vi "Read alarm XML.vi"(11 "模块名称":string) -> (3 "报警输出":string[][](array[string]))   [LabVIEW 2016, in "斯坦道CODMn新电路板.lvlib"]
uses:
  <vilib>/Utility/xml.llb/Write to XML File(string).vi
  <vilib>/Utility/xml.llb/Read From XML File(string).vi
panel:
  in  "报警常量":string[][](array[string])=[["1", "1007", "缺试剂告警", "1、是否缺试剂，及时补充试剂\n2、对应的试剂阀口堵塞，及时清理并更换连接头。\n3、管路气密性不佳\n4、检查传感器与电路板连接、查看传感器光值是否异常"], ["2", "1008", "缺水样告警", "1、配水箱内无水样\n2、对应的水样阀口堵塞或者三通阀坏掉，不能正常切换\n3、往复式注射泵异常，或者管路气密性不佳\n4、检查水样传感器与电路板连接、查看水样传感器光值是否异常"], ["3", "1009", "缺纯水告警", "1、建议排查管路是否异常\n2、供电情况是否正常"], ["4", "1010", "缺标液告警", "1、注射泵水样阀口堵塞；\n2、注射泵阀过载或丝杆无动作。"], ["5", "2007", "仪表漏液告警", "1、建议排查管路是否异常\n2、供电情况是否正常"], ["6", "1011", "标定异常告警", "1、建议排查管路是否异常\n2、供电情况是否正常"], ["7", "4", "超量程告警", "1、建议排查管路是否异常\n2、供电情况是否正常"], ["8", "2008", "加热告警", "检查温度传感器、检查加热片是否损坏或脱落、检查加热模块与电路板接线是否正常、检查固件是否匹配"], ["9", "1051", "低试剂预警", "1、建议排查管路是否异常\n2、供电情况是否正常"], ["10", "1", "超上限告警", "1、建议排查管路是否异常\n2、供电情况是否正常"], ["11", "2", "超下限告警", "1、建议排查管路是否异常\n2、供电情况是否正常"], ["12", "1012", "其他告警", "1、建议排查管路是否异常\n2、供电情况是否正常"], ["13", "1028", "滴定异常告警", "1、配水箱内无水样；\n2、配水箱到模块的管路气密性不佳；\n3、注射泵水样阀口堵塞；\n4、注射泵阀过载或丝杆无动作。"], ["14", "1069", "电极异常告警", "1、建议排查管路是否异常\n2、供电情况是否正常"], ["15", "3", "量程切换告警", "1、建议排查管路是否异常\n2、供电情况是否正常"], ["16", "1070", "参数设置告警", "1、建议排查管路是否异常\n2、供电情况是否正常"], ["17", "1071", "pH电极电位异常", "1、建议排查管路是否异常\n2、供电情况是否正常"], ["18", "1072", "电导率电极异常", "1、建议排查管路是否异常\n2、供电情况是否正常"], ["19", "1073", "浊度光度异常", "1、建议排查管路是否异常\n2、供电情况是否正常"], ["20", "1074", "溶解氧电极异常", "1、建议排查管路是否异常\n2、供电情况是否正常"], ["21", "1029", "缺高锰酸钾告警", "1、建议排查管路是否异常\n2、供电情况是否正常"], ["22", "1030", "缺草酸钠告警", "1、建议排查管路是否异常\n2、供电情况是否正常"], ["23", "1031", "缺硫酸告警", "1、建议排查管路是否异常\n2、供电情况是否正常"], ["24", "1078", "溶解氧异常告警", "1、建议排查管路是否异常\n2、供电情况是否正常"], ["25", "1079", "电导率异常告警", "1、建议排查管路是否异常\n2、供电情况是否正常"], ["26", "1080", "浊度异常告警", "1、建议排查管路是否异常\n2、供电情况是否正常"], ["27", "1081", "叶绿素a异常告警", "1、建议排查管路是否异常\n2、供电情况是否正常"], ["28", "1082", "藻密度异常告警", "1、建议排查管路是否异常\n2、供电情况是否正常"], ["29", "1083", "蓝绿藻异常告警", "1、建议排查管路是否异常\n2、供电情况是否正常"], ["30", "1084", "ORP异常告警", "1、建议排查管路是否异常\n2、供电情况是否正常"], ["31", "1085", "氨氮异常告警", "1、建议排查管路是否异常\n2、供电情况是否正常"], ["32", "1086", "清洁刷异常告警", "1、建议排查管路是否异常\n2、供电情况是否正常"], ["33", "1087", "SD卡异常告警", "1、建议排查管路是否异常\n2、供电情况是否正常"], ["34", "1088", "蓝牙异常告警", "1、建议排查管路是否异常\n2、供电情况是否正常"], ["35", "1089", "WIFI异常告警", "1、建议排查管路是否异常\n2、供电情况是否正常"], ["36", "1013", "缺流程告警", "流程未写入、芯片异常，未存储"], ["37", "1014", "芯片存储异常告警", "固件异常"], ["38", "1015", "缺公式告警", "公式未写入、芯片异常，未存储"], ["39", "1032", "ORP值异常告警", "请检查是否缺水样、ORP电极与电路板连接、更换ORP电极、更换ORP电极采集板，电路板排查"], ["40", "1033", "A值异常告警", "（1）水样浓度过高，需切换到高量程测试。\n（2）缺高锰酸钾或硫酸，可通过试剂报警判断。\n（3）高锰酸钾过期，浓度降低。\n（4）试剂管路或者阀口气密性不好，有空气进入。\n（5）九通注射泵故障，没有正常进样。\n（6）ORP电极故障，无法正常工作。（可通过单步启动测试，观察电极读数有无明显变化）"], ["41", "1034", "B值异常告警", "（1）缺草酸钠或硫酸，可通过试剂报警判断。\n（2）草酸钠过期，浓度降低较多。\n（3）试剂管路或者阀口气密性不好，有空气进入。\n（4）九通注射泵故障，没有正常进样。\n（5）ORP电极故障，无法正常工作。（可通过单步启动测试，观察电极读数有无明显变化）"], ["42", "1035", "环境温度传感器告警", "检查温度传感器与电路板连接，更换温度传感器排查"], ["43", "1036", "注射器保温温度异常告警", "检查温度传感器与电路板连接，更换温度传感器排查"], ["44", "1037", "注射器保温加热超时告警", "检查加热保温圈是否损坏或脱落、加热保温圈与电路板连接、温度传感器是否脱落"], ["96", "1999", "高锰酸钾试剂余量过低，请及时维护", "1、建议排查管路是否异常\n2、供电情况是否正常"], ["97", "1999", "草酸钠试剂余量过低，请及时维护", "1、建议排查管路是否异常\n2、供电情况是否正常"], ["98", "1999", "硫酸试剂余量过低，请及时维护", "1、建议排查管路是否异常\n2、供电情况是否正常"], ["99", "1023", "注射泵配置异常告警", "1、建议排查管路是否异常\n2、供电情况是否正常"], ["103", "1020", "注射泵供电异常告警", "代码103：注射泵未初始化，检查电压是否正常"], ["105", "1021", "注射泵管路阻塞告警", "代码105：检查丝杆是否生锈、检查注射器阻力是否正常、检查注射泵自检是否正常"], ["106", "1022", "注射泵阀头切换过载告警", "代码106：检查阀口是否堵塞、检查多通阀转子接触面是否黏结"], ["250", "1044", "偏心轮运行超时告警", "运行超时告警，检查该器件是否正常运转，或者运转非常缓慢，更换器件排查"], ["253", "1999", "加热温度超限告警", "检查温度传感器与电路板连接、检查是否缺水样"], ["254", "1999", "加热或者降温超时告警", "1、建议排查管路是否异常\n2、供电情况是否正常"], ["255", "1024", "注射泵通讯异常告警", "代码255：检查注射泵与电路板通讯是否正常"]]
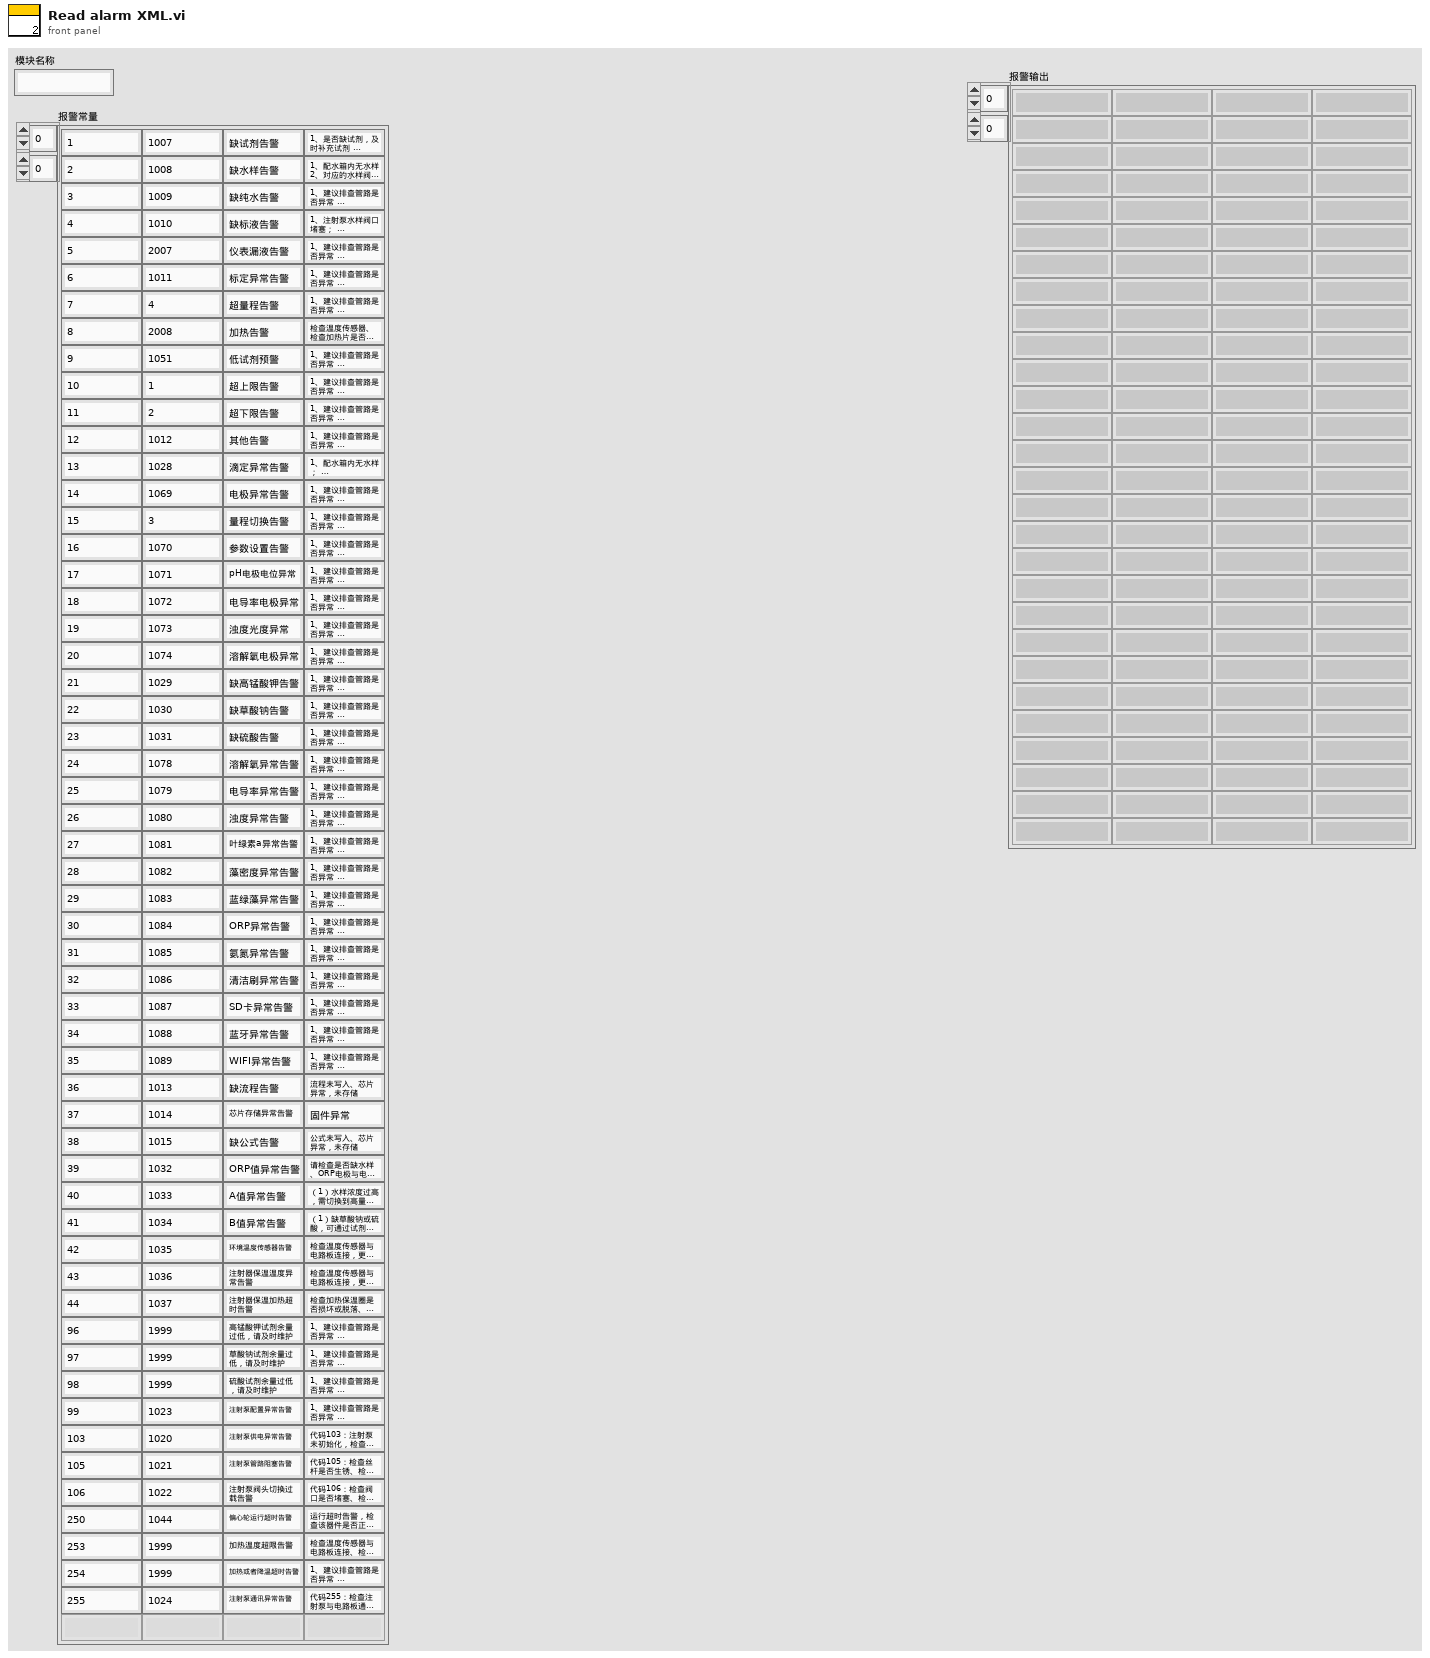
[diagram p1: front panel]
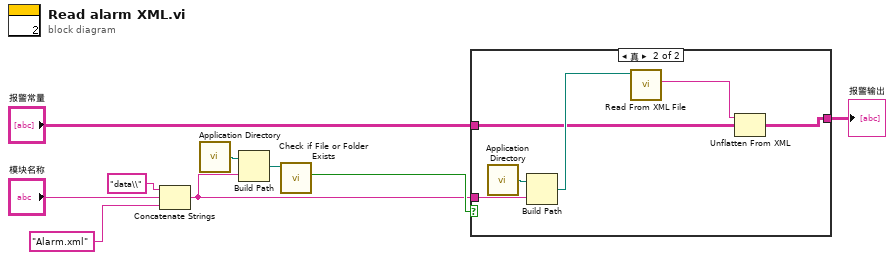
[diagram p0: block diagram]
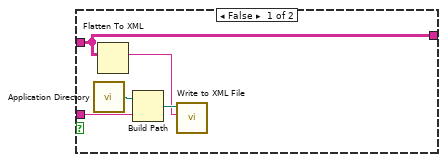
[diagram p2: hidden frame]
diagram:
  n1 = Concatenate Strings("data\\" ("字符串"), "模块名称", "Alarm.xml" ("名称或相对路径")) -> (w6:string)
  n2 = call <vilib>:"Application Directory.vi"() -> ("Application Directory"=w4:path)
  n3 = Build Path(base path=w4, name or relative path=w6) -> (appended path=w5:path)
  n4 = call <vilib>:"Check if File or Folder Exists.vi"("path"=w5) -> ("file or folder exists?"=w7:bool)  [unwired: 8 in, 2 out]
  n5 = case shown="真" w7 {
    tunnel: [w10 w17] -> w8
    tunnel: w6 -> [w11 w16]
    tunnel: "报警常量" -> [w10 w15]
    frame False {
      n6 = call <vilib>:"Application Directory.vi"() -> ("Application Directory"=w13:path)
      n7 = Flatten To XML(anything=w10) -> (xml string=w12:string)
      n8 = Build Path(base path=w13, name or relative path=w11) -> (appended path=w14:path)
      n9 = call-poly <vilib>:"Write to XML File.vi"("XML Input"=w12, "XML File Path"=w14) -> ()  [unwired: 7 in, 3 out]
    }
    frame True {
      n10 = call <vilib>:"Application Directory.vi"() -> ("Application Directory"=w19:path)
      n11 = Build Path(base path=w19, name or relative path=w16) -> (appended path=w18:path)
      n12 = call-poly <vilib>:"Read From XML File.vi"("XML File Path"=w18) -> ("XML Elements"=w20:string)  [unwired: 8 in, 2 out]
      n13 = Unflatten From XML(xml string=w20, type=w15) -> (value=w17:string[][])  [unwired: 1 in, 1 out]
    }
  }
  "报警输出" <- w8
